vi "Disconnect.vi"(3 "error in":errorcluster, 4 "endpoint":string, 5 "socket in":refnum<class "Socket.lvclass">) -> (0 "error out":errorcluster, 2 "socket out":refnum<class "Socket.lvclass">)   [LabVIEW 2025, in "ZeroMQ.lvlib" / "Socket.lvclass"]
doc: "Disconnect the given socket from the specified <b>endpoint</b>. Opposite of zmq_connect. Use zmq_close to disconnect from all endpoints.\n\nDetailed API documentation: http://api.zeromq.org/3-2:zmq-disconnect"
uses:
  Socket.lvclass
  Socket.lvclass/Socket.ctl
  libzmq-v143-mt-4_3_6/LibZMQ.lvlib
panel:
  # "ØMQ"
  # "labview"
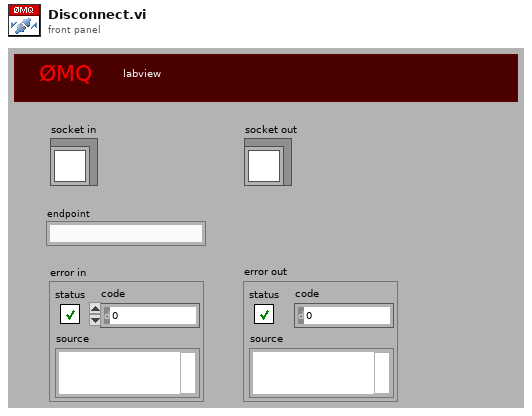
[diagram p1: front panel]
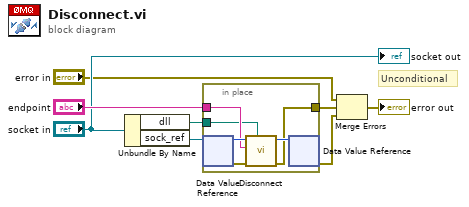
[diagram p0: block diagram]
diagram:
  # "Unconditional"
  n1 = Unbundle By Name("socket in") -> ("dll"=w1:path, "sock_ref"=w5:refnum<data-value>)
  n2 = in-place {
    in-place-border: "endpoint" -> [w13]
    in-place-border: [w10] -> w7
    in-place-border: w1 -> [w9]
    n3 = in-place-dvr #1(w5) -> (w14:u64, w12:errorcluster)
    n4 = call "Disconnect.vi"("path in"=w9, "error in (no error)"=w12, "addr_"=w13, "s_"=w14) -> ("error out"=w10:errorcluster, "s_ out"=w11:u64)  [unwired: 6 in]
    n5 = in-place-dvr #1(w11) -> (w2:errorcluster)  [unwired: 1 out]
  }
  n6 = Merge Errors("error in", w7, w2) -> (→"error out":errorcluster)
  "socket out" <- "socket in"
